vi "Part 1.vi"(11 "Input":string="Game 1: 1 blue, 1 red; 10 red; 8 red, 1 blue, 1 green; 1 green, 5 blue\nGame 2: 9 green, 11 red; 1 green, 7 red, 1 blue; 1 red, 1 blue, 1 green; 11 green, 3 red, 1 blue; 5 green, 12 red; 8 green, 1 blue, 7 red\nGame 3: 16 blue, 2 red, 4 green; 8 red, 4 green; 7 green, 16 blue\nGame 4: 3 green, 4 blue, 6 red; 7 red, 12 green, 5 blue; 5 green, 16 red, 8 blue\nGame 5: 4 green, 4 blue, 3 red; 4 green, 7 red, 1 blue; 2 blue, 2 red, 4 green; 3 green, 7 red, 4 blue; 2 blue, 3 green, 8 red\nGame 6: 3 green, 4 blue, 10 red; 13 red, 3 green, 4 blue; 11 red; 14 red, 1 green; 6 red, 2 green, 1 blue; 10 red, 1 blue, 1 green\nGame 7: 2 green, 9 red, 9 blue; 12 red, 14 blue; 8 red, 3 green\nGame 8: 9 green, 1 red; 18 green, 2 red, 7 blue; 1 blue, 9 green, 3 red; 3 red, 15 blue, 18 green\nGame 9: 2 red, 1 blue, 10 green; 4 red, 1 blue, 5 green; 6 green, 3 red; 1 green, 2 blue; 8 red\nGame 10: 9 green; 6 red, 4 green, 4 blue; 9 red, 2 blue, 9 green; 8 blue, 9 red, 12 green; 4 red, 8 green, 2 blue; 6 green, 7 blue\nGame 11: 1 blue, 15 red, 2 green; 3 green, 9 red; 1 blue, 3 red, 1 green; 10 red, 1 green; 3 red\nGame 12: 6 blue, 9 red, 4 green; 1 green, 8 blue; 4 green, 8 blue, 1 red; 7 green, 7 blue, 2 red\nGame 13: 11 green, 8 blue, 1 red; 5 blue, 2 red, 5 green; 2 red, 18 green; 5 blue, 5 green, 2 red\nGame 14: 1 red, 4 blue, 3 green; 2 red, 1 green, 1 blue; 1 red, 5 green, 1 blue; 3 red, 4 green, 4 blue\nGame 15: 2 blue, 1 green; 3 red, 2 blue, 7 green; 1 red, 4 green, 15 blue; 1 green, 14 blue, 2 red\nGame 16: 3 red, 10 blue, 9 green; 20 blue, 13 green, 1 red; 9 green, 11 blue, 6 red\nGame 17: 4 red, 1 green, 1 blue; 1 green, 1 red, 11 blue; 1 red, 7 blue\nGame 18: 5 red, 9 green; 17 green, 2 blue, 16 red; 11 red, 2 blue, 1 green\nGame 19: 3 red, 14 green; 4 blue, 1 red, 17 green; 14 green, 3 red, 9 blue; 9 blue, 8 green, 8 red; 4 green, 8 blue\nGame 20: 8 green, 3 blue, 3 red; 5 green, 6 red, 1 blue; 1 blue, 6 red, 13 green; 1 blue, 4 red; 4 red, 4 green, 1 blue\nGame 21: 10 green, 3 blue, 7 red; 4 green, 14 blue, 11 red; 2 red, 8 green, 15 blue; 13 green, 7 blue, 4 red\nGame 22: 3 blue, 11 green, 3 red; 7 green, 2 blue, 2 red; 3 red, 3 blue, 15 green; 12 green, 2 blue, 5 red\nGame 23: 4 red, 3 blue; 2 green, 7 red, 6 blue; 1 green, 2 red, 3 blue\nGame 24: 7 red, 3 green, 2 blue; 3 red, 9 green, 9 blue; 8 green, 6 red, 7 blue\nGame 25: 2 red, 2 green, 2 blue; 3 green, 1 red, 4 blue; 4 red, 3 blue; 4 green, 1 blue, 5 red; 2 green, 4 red, 2 blue; 5 green, 3 red\nGame 26: 1 red, 7 blue, 12 green; 2 blue, 2 red, 7 green; 3 green, 5 red, 6 blue; 8 green, 3 blue, 5 red; 15 green, 7 blue\nGame 27: 4 blue, 7 red, 15 green; 4 red, 1 blue, 15 green; 3 red; 8 red, 4 blue, 10 green; 4 red\nGame 28: 2 blue, 5 red, 8 green; 13 red, 9 green; 2 blue, 4 red, 5 green; 1 blue, 14 green, 12 red; 13 green, 11 red, 3 blue\nGame 29: 7 green, 10 red; 9 green, 2 red, 1 blue; 3 blue, 13 green, 5 red\nGame 30: 3 green, 6 blue, 5 red; 3 green, 1 red, 13 blue; 2 red, 2 green, 7 blue; 13 red, 2 green, 9 blue; 2 blue, 7 red, 2 green\nGame 31: 8 red, 16 green, 1 blue; 10 red, 3 blue, 11 green; 2 green, 4 blue, 3 red; 2 blue, 7 red, 12 green; 16 green, 9 red, 6 blue; 8 blue, 9 red, 11 green\nGame 32: 6 red, 3 green, 7 blue; 3 green, 7 blue, 3 red; 4 green, 1 red, 7 blue; 7 blue, 6 green, 5 red; 9 green, 11 red\nGame 33: 8 green, 6 blue; 2 green, 8 red, 1 blue; 12 green, 4 blue, 14 red; 11 blue, 1 green, 7 red; 1 blue, 5 green, 9 red; 7 green, 7 red, 5 blue\nGame 34: 5 blue, 6 green, 7 red; 6 blue, 5 green, 10 red; 9 red, 3 blue, 7 green; 9 red, 4 green; 15 red, 6 green, 4 blue\nGame 35: 6 blue, 4 green, 7 red; 2 blue, 6 red; 4 green, 11 red, 2 blue; 2 red, 1 blue, 4 green; 10 red, 10 blue, 1 green; 11 blue, 4 green\nGame 36: 13 blue, 6 green, 7 red; 5 red, 9 blue, 9 green; 6 red, 2 blue, 3 green; 2 blue, 7 green; 7 red, 5 blue; 12 blue, 7 red, 3 green\nGame 37: 2 red, 12 green, 3 blue; 6 red, 4 blue; 3 blue, 1 green; 4 red, 5 blue, 6 green\nGame 38: 3 red, 16 blue, 10 green; 6 red, 5 green, 5 blue; 7 blue, 12 red, 5 green\nGame 39: 17 red, 4 green, 6 blue; 6 blue, 11 red; 18 red, 3 green, 1 blue; 3 blue, 6 red, 2 green; 19 red, 5 blue\nGame 40: 1 red, 2 green, 3 blue; 6 blue, 5 green, 1 red; 5 green, 1 blue\nGame 41: 7 blue, 6 green; 8 blue, 2 red, 3 green; 2 blue, 3 green; 3 green, 7 red, 17 blue\nGame 42: 6 blue; 10 red, 5 blue, 14 green; 1 blue, 11 green; 6 blue, 2 green, 5 red; 7 blue, 13 green, 11 red\nGame 43: 15 green, 3 blue; 7 blue, 14 green; 11 blue, 3 green; 17 green, 1 red, 1 blue; 17 green, 2 blue, 1 red\nGame 44: 11 red, 4 blue, 16 green; 11 blue, 16 green; 14 red, 10 blue, 17 green\nGame 45: 6 blue; 6 green, 6 blue, 1 red; 5 blue, 11 green; 4 green, 6 blue\nGame 46: 6 green, 3 blue, 2 red; 9 green, 4 red, 2 blue; 9 green, 1 red, 3 blue\nGame 47: 6 red, 3 blue, 9 green; 3 green, 11 blue; 4 blue, 1 red; 11 green, 11 blue\nGame 48: 13 blue, 15 red; 9 red, 9 blue; 15 green, 9 red, 1 blue\nGame 49: 8 green, 4 red; 1 red, 6 blue; 5 blue, 8 green; 1 red, 2 green, 3 blue; 2 red, 5 blue, 5 green\nGame 50: 1 red, 8 green, 3 blue; 1 blue, 9 green; 3 green, 6 blue\nGame 51: 8 green, 8 red, 8 blue; 9 green, 2 red, 6 blue; 1 green, 1 red, 1 blue; 5 blue, 1 red, 7 green; 7 blue, 5 red, 5 green\nGame 52: 2 green, 1 red; 4 blue, 7 red, 2 green; 3 red, 4 blue; 1 green, 1 blue, 7 red; 8 red, 1 green, 8 blue; 4 blue, 3 green, 4 red\nGame 53: 9 blue, 9 red; 3 blue, 3 green, 5 red; 1 green, 6 blue, 2 red; 4 red, 3 green, 3 blue\nGame 54: 1 blue, 2 red, 2 green; 6 green, 1 blue, 3 red; 1 green, 1 blue\nGame 55: 14 red, 8 blue; 9 red, 2 green, 8 blue; 6 blue, 11 red, 1 green; 10 red, 3 blue, 4 green; 13 red, 2 green, 4 blue; 5 green, 5 blue, 3 red\nGame 56: 12 green, 3 blue; 1 red, 13 green, 5 blue; 17 blue, 6 red, 2 green; 4 red, 12 green, 12 blue\nGame 57: 9 green, 9 red, 10 blue; 10 blue, 10 red, 9 green; 4 blue, 14 red, 8 green; 14 red, 7 green; 10 green, 3 blue, 7 red; 1 red, 2 blue, 1 green\nGame 58: 1 green, 9 red, 11 blue; 5 green, 11 red, 6 blue; 2 green, 3 red, 8 blue; 2 green, 14 blue, 4 red; 9 blue, 1 red\nGame 59: 10 blue, 13 green, 3 red; 4 red, 12 green, 8 blue; 4 red, 9 blue, 10 green; 17 green, 5 red, 7 blue; 4 red, 3 blue, 10 green\nGame 60: 4 green; 5 blue, 8 red; 19 red, 3 blue, 2 green; 4 green, 14 blue, 3 red\nGame 61: 2 red, 6 blue; 15 blue, 5 red; 1 green, 2 red; 1 green, 2 blue, 8 red; 7 red, 10 blue; 11 blue\nGame 62: 10 blue, 2 green, 7 red; 2 red, 2 green, 10 blue; 5 red\nGame 63: 19 red; 1 green, 2 blue, 3 red; 1 blue, 11 red\nGame 64: 11 red, 3 green; 3 red, 1 blue, 3 green; 2 green, 2 red, 4 blue; 9 red, 1 green; 3 green, 7 red, 4 blue; 9 red, 2 blue, 3 green\nGame 65: 2 red, 12 green; 3 red, 3 green; 8 green, 1 blue, 4 red; 2 red, 3 green\nGame 66: 4 blue, 11 red, 15 green; 1 blue, 2 green, 10 red; 4 red, 5 green; 16 red, 16 green, 4 blue\nGame 67: 6 red, 1 green; 1 green, 1 blue, 12 red; 11 red, 2 blue\nGame 68: 4 green, 5 red; 9 blue, 1 red; 1 green, 2 red, 7 blue; 6 red, 5 green, 8 blue; 2 green, 7 red, 2 blue\nGame 69: 9 red, 16 green, 12 blue; 5 red, 4 green, 3 blue; 6 green, 11 blue, 6 red; 13 green, 16 blue, 7 red; 1 red, 8 blue, 14 green\nGame 70: 7 red, 5 blue, 4 green; 6 red, 12 blue, 13 green; 5 green, 4 red, 8 blue; 9 blue, 5 green, 2 red\nGame 71: 15 red, 3 green, 3 blue; 1 red, 5 green, 6 blue; 6 green, 7 blue, 16 red\nGame 72: 4 blue, 4 green, 6 red; 9 green, 2 blue; 15 green, 5 red\nGame 73: 1 green, 7 red; 6 red, 2 blue; 5 red, 9 blue; 12 blue, 9 red\nGame 74: 6 blue, 4 red, 4 green; 17 green, 1 blue; 4 blue, 7 green, 4 red\nGame 75: 3 green, 2 blue, 10 red; 17 red, 14 green, 2 blue; 2 green, 1 blue, 14 red; 16 red, 1 blue, 9 green; 14 red, 1 blue, 9 green\nGame 76: 1 red, 10 green, 4 blue; 4 blue, 4 red, 7 green; 1 red, 2 blue, 15 green; 5 blue, 7 green, 1 red; 5 blue, 3 red, 17 green; 18 green, 4 blue, 1 red\nGame 77: 4 green, 5 blue, 7 red; 3 blue, 4 red, 5 green; 1 red, 1 green; 6 green, 4 blue, 16 red\nGame 78: 2 blue, 9 red; 7 red, 3 blue, 18 green; 2 blue, 12 green\nGame 79: 3 red, 10 green, 10 blue; 10 blue, 12 green; 7 green, 10 blue, 3 red\nGame 80: 10 green, 2 blue, 14 red; 3 blue, 4 red; 12 green; 3 red, 2 blue, 1 green; 10 red, 12 green, 2 blue\nGame 81: 1 green, 3 red, 6 blue; 5 blue, 1 red, 1 green; 6 blue, 9 red\nGame 82: 3 blue, 11 red, 20 green; 15 red, 5 green, 3 blue; 4 red, 7 green, 3 blue\nGame 83: 5 red, 12 blue, 6 green; 11 green, 9 blue, 6 red; 6 green, 1 red, 7 blue; 16 blue, 4 red; 3 green, 6 blue\nGame 84: 3 red, 3 blue, 2 green; 3 red, 9 green; 2 blue, 11 green, 1 red; 1 red, 11 green, 1 blue\nGame 85: 11 green, 1 red, 2 blue; 6 red, 8 green, 14 blue; 3 red, 6 green, 15 blue; 9 blue, 7 red, 1 green; 19 blue, 2 green, 5 red; 6 blue, 7 red, 6 green\nGame 86: 11 red, 4 green; 2 green, 1 blue, 10 red; 11 red, 3 blue, 9 green\nGame 87: 2 green, 17 blue; 12 blue, 3 red, 2 green; 3 green, 2 blue, 13 red; 6 red, 3 green; 13 blue, 11 red, 3 green; 5 blue, 7 red, 1 green\nGame 88: 1 red, 12 green; 4 green, 3 blue; 6 blue, 12 green; 1 red, 2 blue\nGame 89: 9 green, 2 red, 12 blue; 19 green, 12 blue, 3 red; 2 red, 8 blue, 11 green; 13 blue, 8 red, 9 green\nGame 90: 2 red, 2 blue, 7 green; 7 green, 2 red, 12 blue; 6 red, 9 green, 5 blue\nGame 91: 14 blue, 2 red, 7 green; 7 blue, 7 green; 1 red, 5 green, 10 blue; 4 red, 7 blue, 4 green; 5 green, 1 red, 13 blue; 5 green, 1 red\nGame 92: 6 green, 4 blue, 7 red; 18 blue, 3 red; 6 red, 2 blue; 16 blue, 5 red, 3 green\nGame 93: 6 red, 17 blue, 5 green; 14 red, 16 blue, 10 green; 11 blue, 7 red, 11 green; 6 blue, 7 green, 3 red; 17 blue, 1 green\nGame 94: 4 green, 9 blue; 2 green, 6 red, 3 blue; 5 red, 4 green, 8 blue; 4 green, 5 red, 6 blue; 7 green, 7 red, 6 blue\nGame 95: 6 blue, 2 red, 3 green; 9 green, 2 blue; 2 red, 4 blue, 11 green; 4 blue, 4 red, 8 green; 13 green, 5 red, 7 blue; 4 red, 15 green, 2 blue\nGame 96: 5 red, 8 blue, 5 green; 12 blue, 2 red; 15 blue, 2 red, 1 green; 4 red, 1 green\nGame 97: 5 red, 5 blue; 1 red, 11 blue; 3 green, 10 blue; 3 green, 1 red, 7 blue; 2 blue, 6 red; 1 red, 1 green, 8 blue\nGame 98: 4 red, 3 blue, 8 green; 5 blue, 2 red, 8 green; 7 green, 10 red, 2 blue; 11 blue, 9 red, 9 green; 6 blue, 10 green, 11 red\nGame 99: 7 green, 3 red, 9 blue; 3 blue, 5 red, 4 green; 2 red, 6 green, 1 blue; 12 blue, 1 red, 1 green; 11 green, 1 red, 12 blue\nGame 100: 2 blue, 1 red; 4 blue, 2 red, 1 green; 7 red, 5 blue; 2 red, 1 green, 5 blue") -> (3 "Output":i64)   [LabVIEW 2021]
uses:
  <userlib>/_OpenG.lib/string/string.llb/Convert EOLs (String)__ogtk.vi
  <vilib>/regexp/Match Regular Expression.xnode
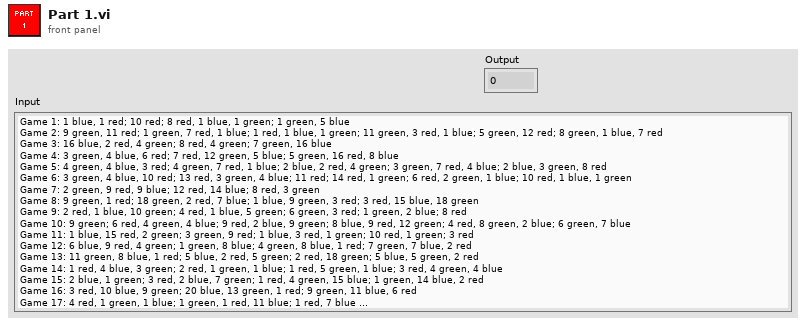
[diagram p1: front panel]
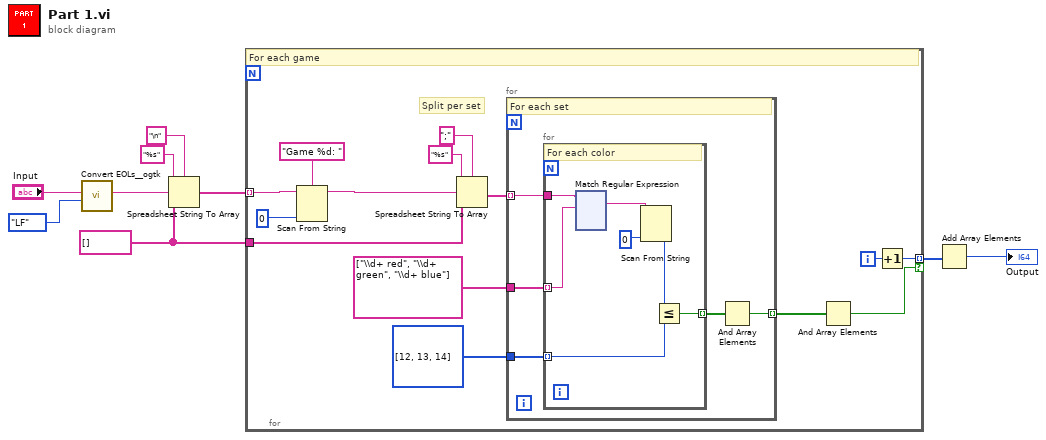
[diagram p0: block diagram]
diagram:
  w4 = string[] []
  n1 = call-poly <userlib>:"Convert EOLs__ogtk.vi"("Convert to:"=enum16{"CR", "LF", "CRLF"}."LF", "String in"="Input") -> ("String out"=w7:string)  [unwired: 9 in]
  n2 = Spreadsheet String To Array(delimiter (Tab)="\n", format string="%s", spreadsheet string=w7, array type (2D Dbl)=w4) -> (array=w5:string[])
  n3 = for {
    tunnel: w5 -> [w23] mode=indexing
    tunnel: w4 -> [w15]
    tunnel: [w12] -> w3 mode=indexing if=w10
    i -> [w13]
    # "Split per set"
    # "For each game"
    n4 = Scan From String(format string="Game %d: ", input string=w23, default 1=0) -> (remaining string=w17:string)  [unwired: 3 in, 2 out]
    n5 = Spreadsheet String To Array(delimiter (Tab)=";", format string="%s", spreadsheet string=w17, array type (2D Dbl)=w15) -> (array=w16:string[])
    n6 = for {
      tunnel: string[] ["\\d+ red", "\\d+ green", "\\d+ blue"] -> [w28]
      tunnel: w16 -> [w27] mode=indexing
      tunnel: i32[] [12, 13, 14] -> [w26]
      tunnel: [w24] -> w11 mode=indexing
      # "For each set"
      n7 = for {
        tunnel: w27 -> [w35]
        tunnel: w28 -> [w32] mode=indexing
        tunnel: w26 -> [w31] mode=indexing
        tunnel: [w29] -> w25 mode=indexing
        # "For each color"
        n8 = xnode "Match Regular Expression"("input string"=w35, "regular expression"=w32) -> ("whole match"=w34:string)  [unwired: 4 in, 4 out]
        n9 = Scan From String(input string=w34, default 1=0) -> (output 1=w30:i32)  [unwired: 3 in, 3 out]
        n10 = Less Or Equal?(x=w30, y=w31) -> (x <= y?=w29:bool)
      }
      n11 = And Array Elements(Boolean array=w25) -> (logical AND=w24:bool)
    }
    n12 = And Array Elements(Boolean array=w11) -> (logical AND=w10:bool)
    n13 = Increment(x=w13) -> (x+1=w12:i32)
  }
  n14 = Add Array Elements(numeric array=w3) -> (sum=→"Output":i32)
